vi "General Server.vi"(11 "DVR In":refnum<data-value>) -> (3 "FPGA Session out":refnum<class "FPGA Session.lvclass">)   [LabVIEW 2016]
uses:
  Session/Raw FPGA/FPGA Session.lvclass
  C:/Program Files (x86)/National Instruments/LabVIEW 2016/vi.lib/MSR Consulting, LLC/General Reuse/Session APIs/_Session Fwk/Session - Root.lvclass
  Data/Nicholas Data.lvclass
  <vilib>/Platform/TimedLoop/XDataNode/timing_clust.ctl
  <vilib>/Platform/TimedLoop/XDataNode/nitl_modes.ctl
  <vilib>/Platform/TimedLoop/XDataNode/wakeup.ctl
  Data/Nicholas Data.lvclass/Nicholas Data.ctl
  Session/Raw FPGA/FPGA Session.lvclass/FPGA Session.ctl
  do bit control.ctl
  Data/Read PAS.vi
  Data/Read CRDS.vi
  Data/Read PPT Data.vi
  Data/Read TE Data.vi
  Data/Read Vaisala Data.vi
  Data/Read Alicat Data.vi
  Session/Raw FPGA/Read FPGA Ref.vi
  <vilib>/Utility/error.llb/Error Cluster From Error Code.vi
  <vilib>/rvi/errors/niLvFpgaAdjustHostInterfaceError.vi
  <vilib>/Platform/TimedLoop/XDataNode/XDataNode.xnode
  <vilib>/MSR Consulting, LLC/General Reuse/PAS/Data/Main/PAS Data.lvclass
  <vilib>/MSR Consulting, LLC/General Reuse/CRDS/Data/Main/CRDS Data.lvclass
  <vilib>/MSR Consulting, LLC/General Reuse/Data/Array Data/Single 1-D/Single_Array.lvclass
  <vilib>/MSR Consulting, LLC/Devices/TE Tech/Data/TECData.lvclass
  <vilib>/MSR Consulting, LLC/Devices/Alicats/Data/Alicat Data.lvclass
  FPGA Ref.ctl
  <vilib>/rvi/interface/nirviReadWriteControl/nirviReadWriteControl.xnode
  FPGA Bitfiles/NickIO.lvbitx
  <vilib>/Platform/TimedLoop/XDataNode/XDNodeRunTimeDep.lvlib
  <vilib>/MSR Consulting, LLC/General Reuse/Session APIs/_Session Fwk/Session - Root.lvclass
  NiFpgaLv.dll
panel:
  out "hex integer string":string
  out "error out":errorcluster
  out "HK Data":fxp<+/-,16,5>[](array[numeric])
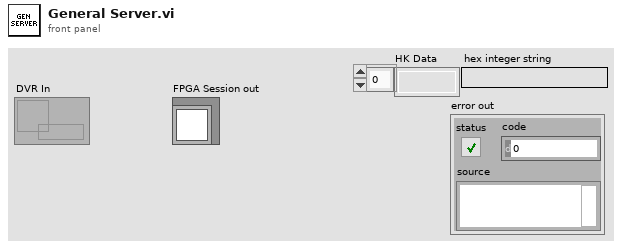
[diagram p1: front panel]
types:
  T1 = typedef "Session - Root.lvclass/Session Handle.ctl" = refnum<data-value>
  T2 = typedef "XDNodeRunTimeDep.lvlib/timing_clust.ctl" = cluster{"Expected End [f-1]":u64, "Actual End [f-1]":u64, "Finished Late? [f-1]":bool, "Expected End [i-1]":u64, "Actual End [i-1]":u64, "Finished Late? [i-1]":bool, "Expected Start [i]":u64, "Actual Start [i]":u64, "Expected Start [f]":u64, "Actual Start [f]":u64, "Source Name":string, "Structure Name":string, "Period":i64, "Deadline":i64, "Offset":i64, "Start":i64, "Priority":i32, "Timeout":i32, "Mode":T3, "Wakeup Reason":T4, "Error":errorcluster, "Source Type":string, "Secondary Source Type":string, "Global End Time":u64, "Global Start Time":u64, "Frame Duration":u64, "Iteration Duration":u64, "Assigned CPU":i32, "I/O Scan Engine Mode":u32}
  T3 = typedef "XDNodeRunTimeDep.lvlib/nitl_modes.ctl" = enum32{"No Change", "Process missed periods, maintain original phase", "Discard missed periods, maintain original phase", "Process missed periods, ignore original phase", "Discard missed periods, ignore original phase"}
  T4 = typedef "XDNodeRunTimeDep.lvlib/wakeup.ctl" = enum32{"Normal", "Aborted", "Asynchronous wakeup", "Timing source error", "Timed loop error", "Timeout"}
  T5 = typedef "do bit control.ctl" = enum16{"uv light ctl 1", "uv light ctl 2", "uv enable", "laser enable", "pas speaker", "compressore enable", "vacuum pump", "o3 add", "scrubber test", "presaure meas 1", "preasure meas 2", "hb ctl 1", "hb ctl 2", "crd laser enable", "pmt enable", "fan enable"}
  T6 = typedef "FPGA Ref.ctl" = refnum<k20>
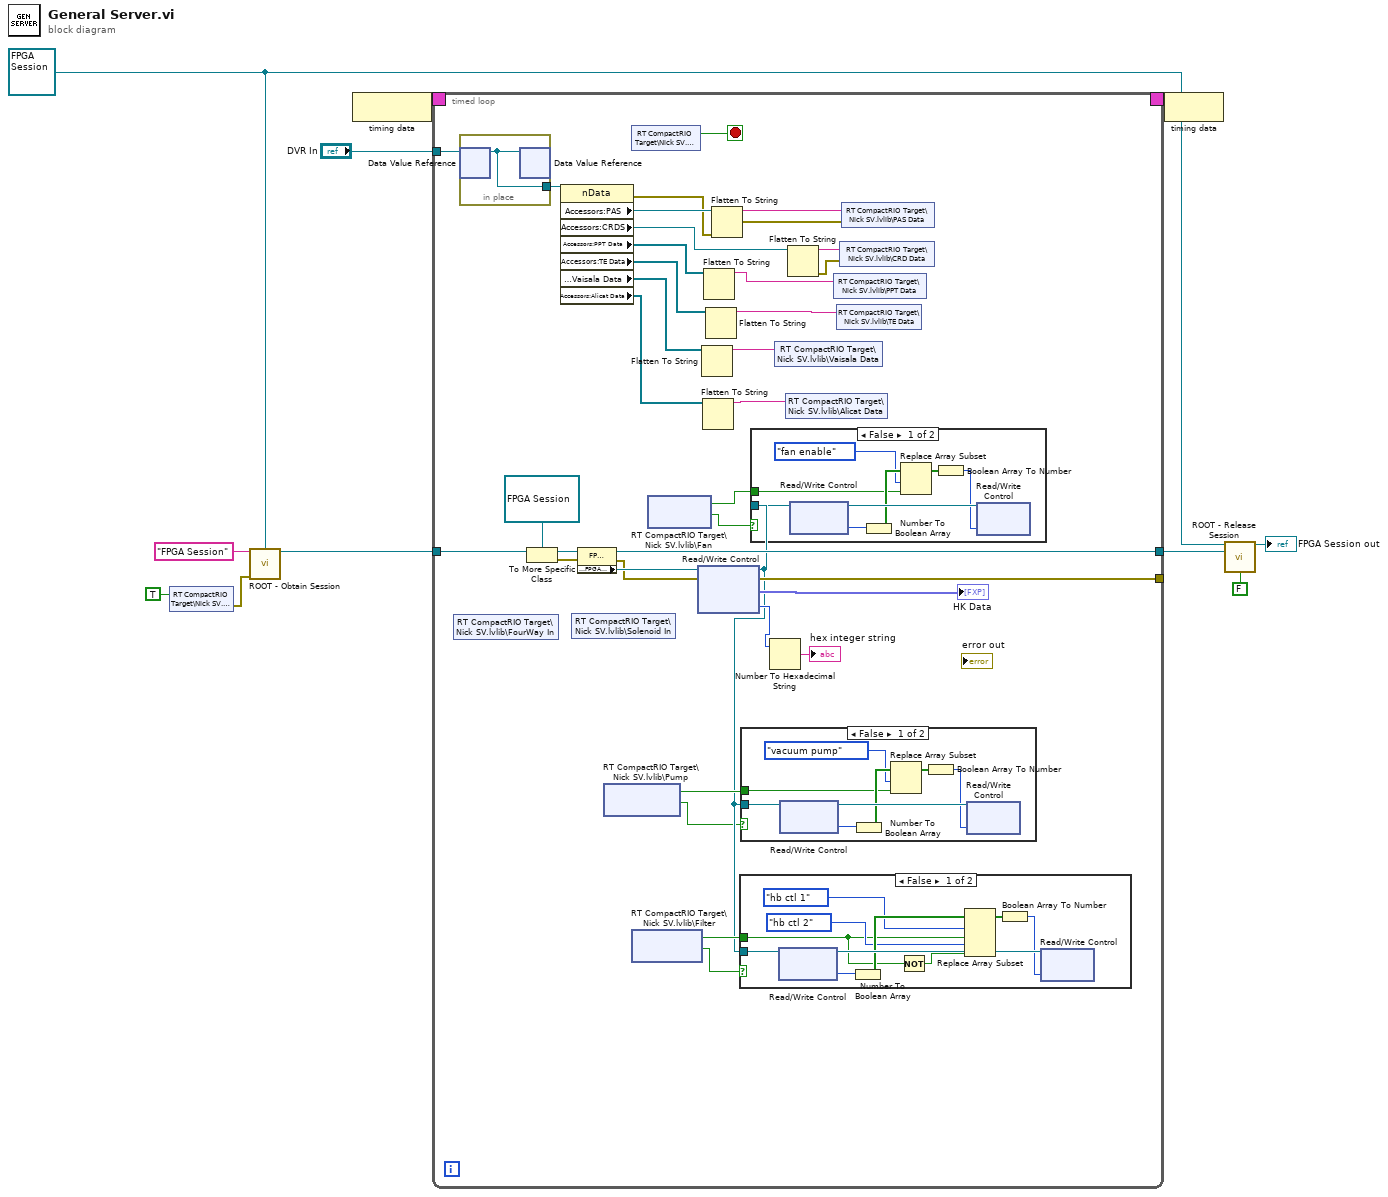
[diagram p0: block diagram]
diagram:
  w9 = refnum<class "FPGA Session.lvclass"> refnum ("FPGA Session")
  n1 = shared-variable "RT CompactRIO Target\\Nick SV.lvlib\\Fan"(TRUE ("Fan")) -> (error out=w1:errorcluster)  [unwired: 1 in]
  n2 = call <vilib>:"ROOT - Obtain Session.vi"("Session Name ()"="FPGA Session", "OBJ - Session"=w9, "error in (no error)"=w1) -> ("Session Handle"=w4:T1)  [unwired: 10 in, 2 out]
  n3 = node-c288() -> (w11:T2)
  n4 = timed-loop {
    timing: w11 -> [_]
    timing-out: [_] -> w10
    tunnel: w4 -> [w46]
    tunnel: [w43] -> w5
    tunnel: "DVR In" -> [w40]
    tunnel: [w24] -> _
    stop <- w47 stop-if-true
    n5 = shared-variable "RT CompactRIO Target\\Nick SV.lvlib\\FourWay In"() -> ()  [unwired: 1 in, 2 out]
    n6 = in-place {
      in-place-border: [w74] -> w36
      n7 = in-place-dvr #1(w40) -> (w74:refnum<class "Nicholas Data.lvclass">)  [unwired: 1 out]
      n8 = in-place-dvr #1(w74) -> ()  [unwired: 2 out]
    }
    n9 = To More Specific Class(target class=refnum<data-value> refnum ("Session Handle"), reference=w46) -> (specific class reference=w44:refnum<data-value>, error out=w39:errorcluster)  [unwired: 1 in]
    n10 = property class="nData"(reference=w36) -> (error out=w32:errorcluster, "Accessors:PAS"=w35:refnum<class "PAS Data.lvclass">, "Accessors:CRDS"=w34:refnum<class "CRDS Data.lvclass">, "Accessors:PPT Data"=w30:refnum<class "Single_Array.lvclass">[], "Accessors:TE Data"=w29:refnum<class "TECData.lvclass">[], "Accessors:Vaisala Data"=w28:refnum<class "Single_Array.lvclass">[], "Accessors:Alicat Data"=w22:refnum<class "Alicat Data.lvclass">[])  [unwired: 1 in, 1 out]
    n11 = shared-variable "RT CompactRIO Target\\Nick SV.lvlib\\Solenoid In"() -> ()  [unwired: 1 in, 2 out]
    n12 = property class="FPGA Session"(reference=w44, error in=w39) -> (reference out=w43:refnum<data-value>, error out=w37:errorcluster, "Accessors:FPGA Ref"=w42:T6)
    n13 = shared-variable "RT CompactRIO Target\\Nick SV.lvlib\\Pump"() -> (w16:bool, w12:bool)  [unwired: 2 in, 1 out]
    n14 = shared-variable "RT CompactRIO Target\\Nick SV.lvlib\\Stop"() -> (w47:bool)  [unwired: 1 in, 1 out]
    n15 = shared-variable "RT CompactRIO Target\\Nick SV.lvlib\\Filter"() -> (w15:bool, w13:bool)  [unwired: 2 in, 1 out]
    n16 = shared-variable "RT CompactRIO Target\\Nick SV.lvlib\\Fan"() -> (w17:bool, w18:bool)  [unwired: 2 in, 1 out]
    n17 = xnode "Read/Write Control"("FPGA VI Reference In"=w42, "error in"=w37) -> ("FPGA VI Reference Out"=w14:T6, "error out"=w24:errorcluster, "HK Data"=→"HK Data":fxp<+/-,16,5>[], "Version"=w20:i64)
    n18 = Flatten To String(anything=w28) -> (data string=w27:string)  [unwired: 3 in, 2 out]
    n19 = Flatten To String(anything=w22) -> (data string=w21:string)  [unwired: 3 in, 2 out]
    n20 = Flatten To String(anything=w30) -> (data string=w26:string)  [unwired: 3 in, 2 out]
    n21 = Flatten To String(anything=w29) -> (data string=w25:string)  [unwired: 3 in, 2 out]
    n22 = Flatten To String(anything=w35, error in (no error)=w32) -> (data string=w41:string, error out=w38:errorcluster)  [unwired: 2 in, 1 out]
    n23 = case shown="False" w13 {
      tunnel: w14 -> [w57 _]
      tunnel: w15 -> [w49 _]
      frame False {
        n24 = xnode "Read/Write Control"("FPGA VI Reference In"=w57) -> ("FPGA VI Reference Out"=w56:T6, "DO Out"=w55:u16)  [unwired: 1 in, 1 out]
        n25 = Number To Boolean Array(number=w55) -> (Boolean array=w54:bool[])
        n26 = Not(x=w49) -> (.not. x?=w48:bool)
        n27 = Replace Array Subset(array=w54, new element #1=w49, index #1=do_bit_control."hb ctl 1" ("Enum"), new element #2=w48, index #2=do_bit_control."hb ctl 2" ("Enum")) -> (w52:bool[])
        n28 = Boolean Array To Number(Boolean array=w52) -> (number=w51:u16)
        n29 = xnode "Read/Write Control"("FPGA VI Reference In"=w56, "DO In"=w51) -> ()  [unwired: 1 in, 2 out]
      }
      frame True {
      }
    }
    n30 = case shown="False" w12 {
      tunnel: w14 -> [w65 _]
      tunnel: w16 -> [w60 _]
      frame False {
        n31 = xnode "Read/Write Control"("FPGA VI Reference In"=w65) -> ("FPGA VI Reference Out"=w64:T6, "DO Out"=w63:u16)  [unwired: 1 in, 1 out]
        n32 = Number To Boolean Array(number=w63) -> (Boolean array=w62:bool[])
        n33 = Replace Array Subset(array=w62, new element=w60, index=do_bit_control."vacuum pump" ("Enum")) -> (w59:bool[])
        n34 = Boolean Array To Number(Boolean array=w59) -> (number=w58:u16)
        n35 = xnode "Read/Write Control"("FPGA VI Reference In"=w64, "DO In"=w58) -> ()  [unwired: 1 in, 2 out]
      }
      frame True {
      }
    }
    n36 = case shown="False" w18 {
      tunnel: w14 -> [w66 _]
      tunnel: w17 -> [w69 _]
      frame False {
        n37 = xnode "Read/Write Control"("FPGA VI Reference In"=w66) -> ("FPGA VI Reference Out"=w73:T6, "DO Out"=w72:u16)  [unwired: 1 in, 1 out]
        n38 = Number To Boolean Array(number=w72) -> (Boolean array=w71:bool[])
        n39 = Replace Array Subset(array=w71, new element=w69, index=do_bit_control."fan enable" ("Enum")) -> (w68:bool[])
        n40 = Boolean Array To Number(Boolean array=w68) -> (number=w67:u16)
        n41 = xnode "Read/Write Control"("FPGA VI Reference In"=w73, "DO In"=w67) -> ()  [unwired: 1 in, 2 out]
      }
      frame True {
      }
    }
    n42 = Number To Hexadecimal String(2:w20) -> (0:→"hex integer string":string)  [unwired: 1 in]
    n43 = shared-variable "RT CompactRIO Target\\Nick SV.lvlib\\Vaisala Data"(w27) -> ()  [unwired: 1 in, 1 out]
    n44 = shared-variable "RT CompactRIO Target\\Nick SV.lvlib\\Alicat Data"(w21) -> ()  [unwired: 1 in, 1 out]
    n45 = Flatten To String(anything=w34) -> (data string=w33:string, error out=w31:errorcluster)  [unwired: 3 in, 1 out]
    n46 = shared-variable "RT CompactRIO Target\\Nick SV.lvlib\\PPT Data"(w26) -> ()  [unwired: 1 in, 1 out]
    n47 = shared-variable "RT CompactRIO Target\\Nick SV.lvlib\\TE Data"(w25) -> ()  [unwired: 1 in, 1 out]
    n48 = shared-variable "RT CompactRIO Target\\Nick SV.lvlib\\CRD Data"(w33, error in=w31) -> ()  [unwired: 1 out]
    n49 = shared-variable "RT CompactRIO Target\\Nick SV.lvlib\\PAS Data"(w41, error in=w38) -> ()  [unwired: 1 out]
  }
  n50 = node-c288(w10) -> ()
  n51 = call <vilib>:"ROOT - Release Session.vi"("OBJ - Session in"=w9, "Session Handle in"=w5, "force destroy? (F)"=FALSE) -> ("OBJ - Session out"=→"FPGA Session out":refnum<class "FPGA Session.lvclass">)  [unwired: 11 in, 1 out]
